vi "获取128X4差损.vi"(6 "testType":string, 7 "ref":bool=TRUE, 8 "error in (no error)":errorcluster, 9 "COM":i32, 11 "A":i32) -> (0 "error out":errorcluster, 2 "S21":dbl[][](array[numeric]))   [LabVIEW 2015]
uses:
  Database_util/Ctl/database_Method.ctl
  network_Global/Global.vi
panel:
  out "搜索结果":i32
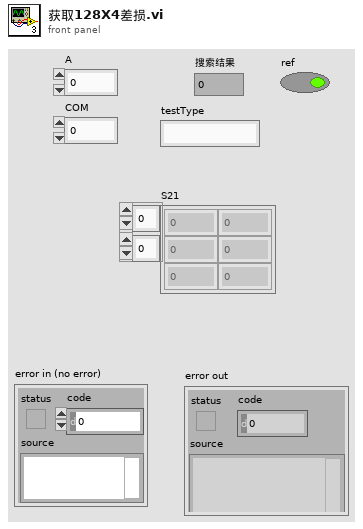
[diagram p1: front panel]
types:
  T1 = typedef "database_Method.ctl" = enum16{"初始化", "查询", "关闭"}
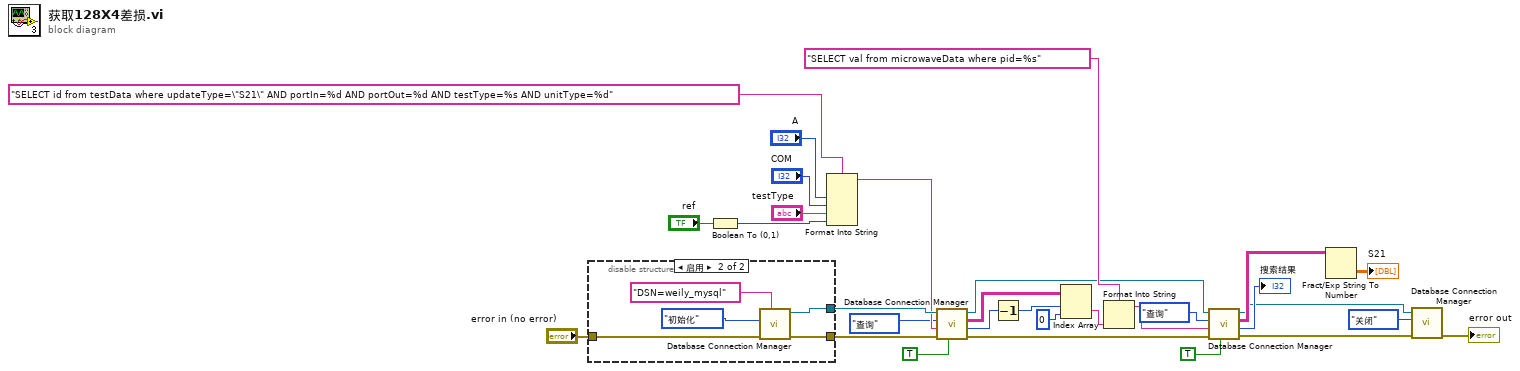
[diagram p0: block diagram]
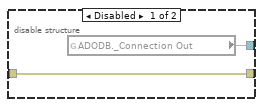
[diagram p2: hidden frame]
diagram:
  n1 = disable-structure shown="启用" {
    disable-tunnel: [w32 w36] -> w21
    disable-tunnel: "error in (no error)" -> [w31 w35]
    disable-tunnel: [w31 w34] -> w11
    frame Disabled {
      n2 = global read "Global.vi" "ADODB._Connection Out"() -> (w32:refnum<k7>)
    }
    frame Enabled {
      n3 = call "Database Connection Manager.vi"("ConnectionString"="DSN=weily_mysql", "error in (no error)"=w35, "Method"=database_Method."初始化") -> ("error out"=w34:errorcluster, "ADODB._Connection Out"=w36:refnum<k7>)  [unwired: 5 in, 2 out]
    }
  }
  n4 = Boolean To (0,1)(Boolean="ref") -> (0, 1=w9:i16)
  n5 = Format Into String(format string="SELECT id from testData where updateType=\"S21\" AND portIn=%d AND portOut=%d AND testType=%s AND unitType=%d" ("SQL"), "A", "COM", "testType", w9) -> (resulting string=w20:string)  [unwired: 2 in, 1 out]
  n6 = call "Database Connection Manager.vi"("Return Data (T)"=TRUE, "error in (no error)"=w11, "Command Text"=w20, "Method"=database_Method."查询", "ADODB._Connection In"=w21) -> ("error out"=w17:errorcluster, "Rows Fetched"=w18:i32, "Data"=w19:string[][], "ADODB._Connection Out"=w16:refnum<k7>)  [unwired: 3 in]
  n7 = Decrement(x=w18) -> (x-1=w29:i32)
  n8 = Index Array(array=w19, index (row)=w29, index (col)=0 ("disabled index (col)")) -> (element=w27:string)
  n9 = Format Into String(format string="SELECT val from microwaveData where pid=%s" ("String"), w27) -> (resulting string=w15:string)  [unwired: 2 in, 1 out]
  n10 = call "Database Connection Manager.vi"("Return Data (T)"=TRUE, "error in (no error)"=w17, "Command Text"=w15, "Method"=database_Method."查询", "ADODB._Connection In"=w16) -> ("error out"=w2:errorcluster, "Rows Fetched"=→"搜索结果":i32, "Data"=w8:string[][], "ADODB._Connection Out"=w1:refnum<k7>)  [unwired: 3 in]
  n11 = Fract/Exp String To Number(string=w8) -> (number=→"S21":dbl[][])  [unwired: 3 in, 1 out]
  n12 = call "Database Connection Manager.vi"("error in (no error)"=w2, "Method"=database_Method."关闭", "ADODB._Connection In"=w1) -> ("error out"=→"error out":errorcluster)  [unwired: 5 in, 3 out]
